vi "Get theme path.vi"(8 "error in":errorcluster, 11 "Theme Config in":refnum<class "Theme Config.lvclass">) -> (0 "error out":errorcluster, 2 "theme path":path, 3 "Theme Config out":refnum<class "Theme Config.lvclass">)   [LabVIEW 2021, in "Theme Config.lvclass"]
uses:
  Theme Config.lvclass
  Theme Config.lvclass/Theme Config.ctl
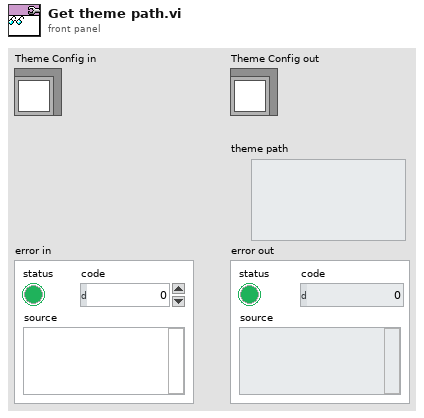
[diagram p1: front panel]
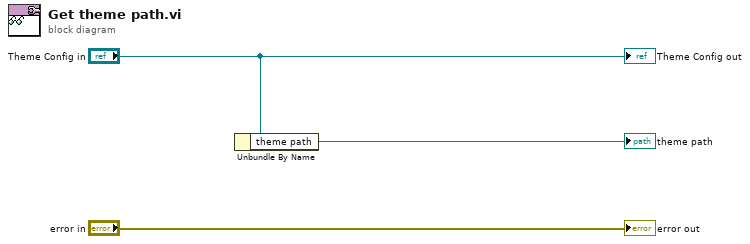
[diagram p0: block diagram]
diagram:
  n1 = Unbundle By Name("Theme Config in") -> ("theme path"=→"theme path":path)
  "error out" <- "error in"
  "Theme Config out" <- "Theme Config in"
